vi "Client Data Display.vi"() -> ()   [LabVIEW 2019]
doc: "The Advanced Serial Read and Write example performs a Serial Port Read, a Serial Port Write, or a combination of these actions while setting some advanced serial features like buffer size, termination characters, and XON/XOFF flow control. The user selects the actions (read or write) on the front panel. If both are selected, the VI will write the data first, read the data and then close the VISA session that is opened to the port. \n\nThe parameters set for the serial port must match the parameters of the connected instrument or device. In this example, the bytes to read parameter specifies the number of bytes that the serial port reads. If there were more bytes at the port than the number specified in bytes to read, those bytes would not be read. Also, if you specify to read more bytes than the number of bytes actually read, you might receive a timeout error message.\n\nINSTRUCTIONS:\n1) Select the serial resource and configuration parameters (baud rate, data bits, parity, stop bits, flow control).\n2) Termination character can be enabled and set. Also, set the required input buffer size prior to running the example.\n3) Select the operations to be performed. \n4) Connect the serial port to your device. If no device is available, perform a loopback test by doing one of the following. Short pins 2 and 3 on a RS-232 cable or short pin 4 to pin 8 and pin 5 to pin 9 on a RS-485/422 cable. \n5) Run the VI to see the data read. (The \"read string\" will match the \"string to write\" if a loopback test was performed.)\n\nThis example exposes several advanced features that you may need for your application. Not all applications need all the features shown in this example. The input buffer size is likely an important setting that you want to control in your application. This example expands upon the flow control option for XON and XOFF, allowing the user to choose those control characters. The timeout parameter has been brought to the front panel so a user can specify the time period the VISA Read will wait for the number of bytes to read before timing out. Also, the user has several controls for the termination character, which is discussed later.\n\nNote that you can press the write and read buttons and change the bytes to read parameters on the fly, while the example is running. However, you must stop the example to change the other configuration parameters after the example has started running, and then run again.\n\nSet the I/O buffer size slightly higher the amount of data you expect to receive. This is very important for applications that don't use flow control, as you may lose characters if the receive buffer overflows.\n\nSetting the timeout period ensures that the operation returns with a timeout error if the operation cannot be performed in the specified time period. \n\nSome devices require a termination character in order to identify the end of command strings. Some devices send a termination character to signify the end of data to be read. \n\nThis example shows how you can end the Read operation once a termination character is detected in the buffer and/or append a termination character at the end of the Write data. To enable the Read to end on a termination character, use the VISA Configure Serial Port or use the VISA Properties Serial End Mode for Reads, Termination Character Enable, and Termination Character. To end the Write with a termination character, use the VISA Properties Serial End Mode for Writes, the Send End Enable, and Termination Character. In this example, the same termination character is used for both the Read and the Write. You can specify two different characters for your application, if desired.\n\nYour application may require specific characters for the XON/XOFF Flow Control. You can specify these characters with the VISA Properties Flow Control XOFF Character and Flow Control XON Character. Note that if the standard XON and XOFF characters are used, then decimal 17 and 19 are unavailable for data values. Remember that using flow control and setting an adequate buffer size allow you to prevent buffer overflows."
uses:
  <vilib>/Instr/_visa.llb/VISA Configure Serial Port (Instr).vi
panel:
  out "Output Data":string
  out "Humidity Chart":dbl(graph)
  out "Temperature Chart":dbl(graph)
  out "Humidity":dbl
  out "Temperature":dbl
  out "Actual Bytes Read":u32=47
  in  "Bytes to Read":u32=100
  in  "Stop":bool
  in  "Parity":u16
  in  "Data Bits":u16=8 min=5 max=8 step=1
  in  "Stop Bits":u16=10
  in  "Baud Rate":u32=115200
  in  "VISA Resource Name":refnum<visa-resource-name>="COM10"
  # "Server Serial Port"
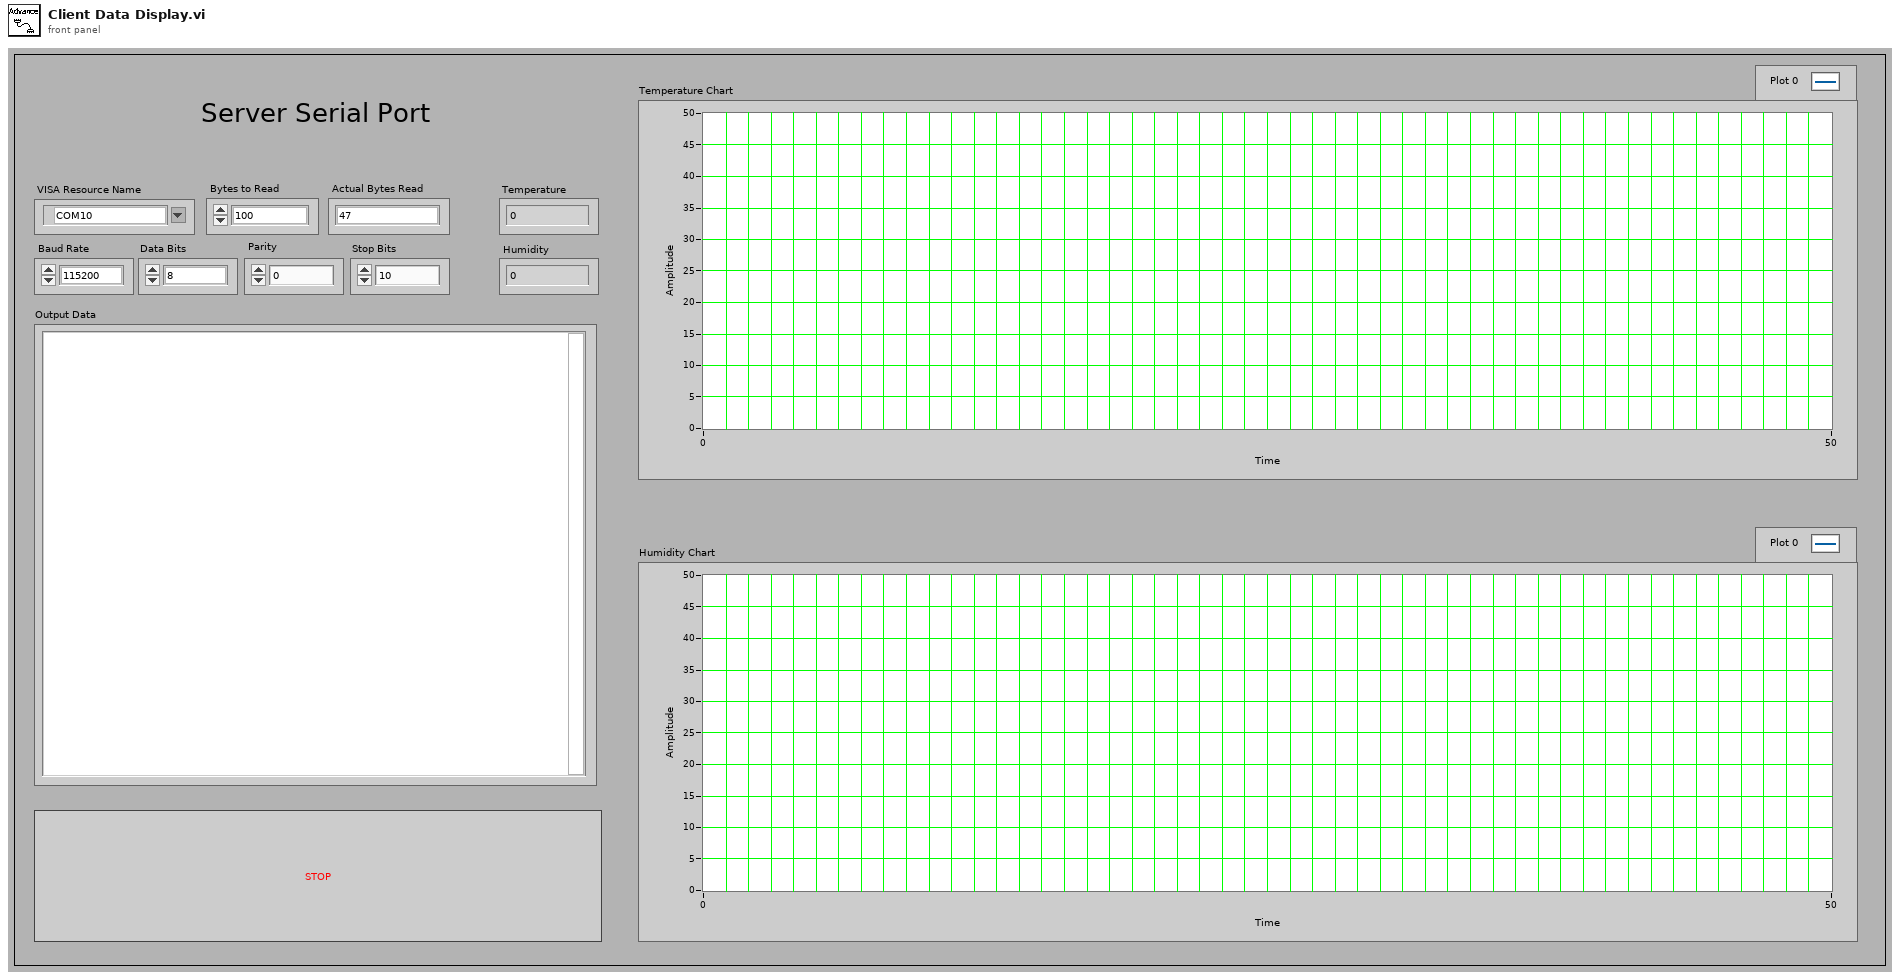
[diagram p1: front panel]
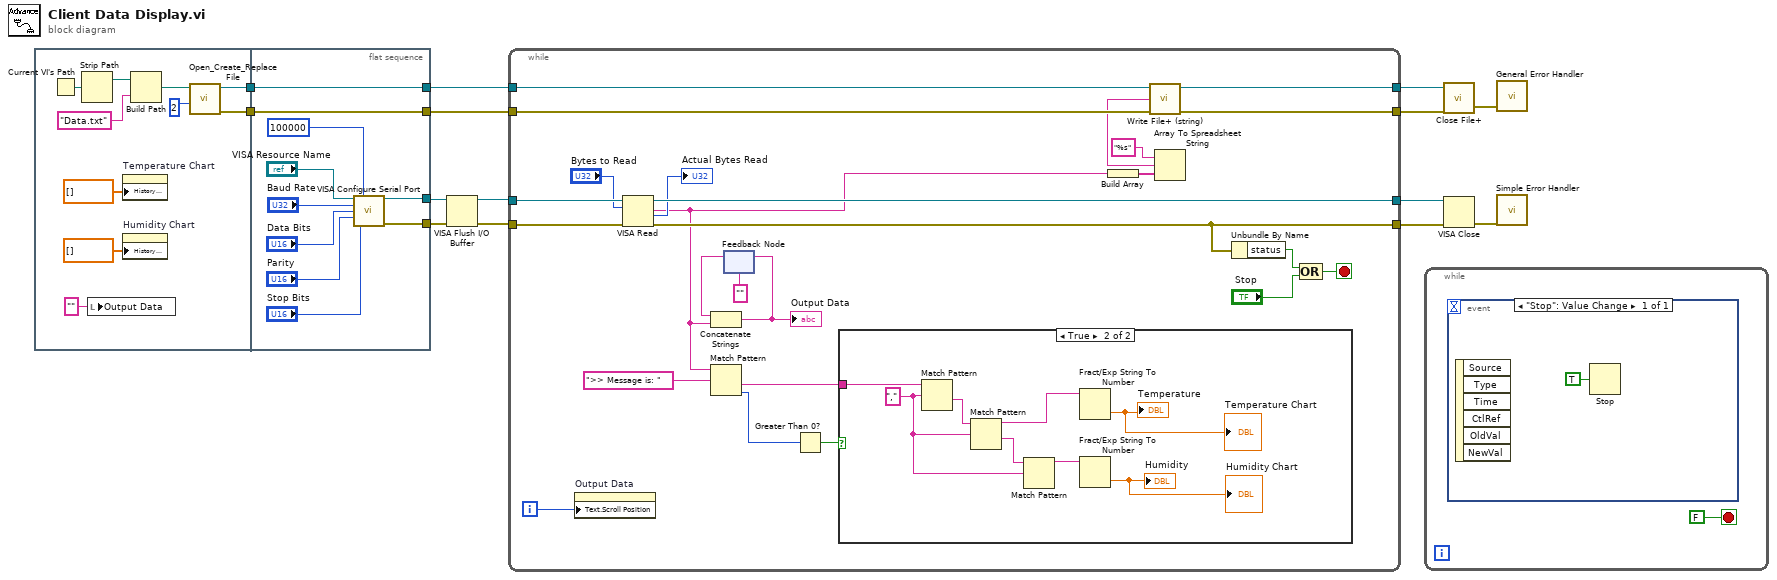
[diagram p0: block diagram]
diagram:
  n1 = flat-sequence {
    tunnel: [w23] -> w6
    tunnel: [w22] -> w5
    tunnel: [w33] -> w9
    tunnel: [w34] -> w10
    tunnel: w6 -> [w34]
    tunnel: w5 -> [w33]
    tunnel: [w27] -> w4
    tunnel: [w26] -> w1
    frame #0 {
      n2 = Current VI's Path() -> (path=w21:path)
      n3 = Strip Path(path=w21) -> (stripped path=w20:path)  [unwired: 1 out]
      n4 = local write "Output Data"("" ("Output Data")) -> ()
      n5 = property on="Temperature Chart" class="WFChart (strict)"("History Data"=dbl[] []) -> ()  [unwired: 2 in, 2 out]
      n6 = property on="Humidity Chart" class="WFChart (strict)"("History Data"=dbl[] []) -> ()  [unwired: 2 in, 2 out]
      n7 = Build Path(base path=w20, name or relative path="Data.txt") -> (appended path=w18:path)
      n8 = call <vilib>:"Open_Create_Replace File.vi"("function (open:0)"=2, "file path"=w18) -> ("error out"=w22:errorcluster, "refnum"=w23:refnum<file>)  [unwired: 4 in, 4 out]
    }
    frame #1 {
      n9 = call-poly "VISA Configure Serial Port"("VISA resource name"="VISA Resource Name", "timeout (10sec)"=u32 100000, "baud rate (9600)"="Baud Rate", "data bits (8)"="Data Bits", "parity (0:none)"="Parity", "stop bits (10: 1 bit)"="Stop Bits") -> ("VISA resource name out"=w27:refnum<visa-resource-name>, "error out"=w26:errorcluster)  [unwired: 4 in, 4 out]
    }
  }
  n10 = VISA Flush I/O Buffer(VISA resource name=w4, error in (no error)=w1) -> (VISA resource name out=w3:refnum<visa-resource-name>, error out=w2:errorcluster)  [unwired: 1 in]
  n11 = while {
    tunnel: w2 -> [w57]
    tunnel: w3 -> [w56]
    tunnel: [w59] -> w13
    tunnel: [w58] -> w12
    tunnel: w10 -> [w50]
    tunnel: w9 -> [w49]
    tunnel: [w51] -> w8
    tunnel: [w52] -> w7
    i -> [w35]
    stop <- w54 stop-if-true
    n12 = property on="Output Data" class="Str"("Text.Scroll Position"=w35) -> ()  [unwired: 2 in, 2 out]
    n13 = VISA Read(VISA resource name=w56, byte count="Bytes to Read", error in (no error)=w57) -> (VISA resource name out=w59:refnum<visa-resource-name>, read buffer=w38:string, return count=→"Actual Bytes Read":u32, error out=w58:errorcluster)
    n14 = Match Pattern(string=w38, regular expression=">> Message is: ") -> (after substring=w39:string, offset past match=w36:i32)  [unwired: 1 in, 2 out]
    n15 = feedback #1("") -> (w46:string)
    n16 = Concatenate Strings(w46, w38) -> (w44:string)
    "Output Data" <- w44
    n17 = feedback-in #1(w44) -> ()
    n18 = Greater Than 0?(x=w36) -> (x > 0?=w37:bool)
    n19 = case shown="True" w37 {
      tunnel: w39 -> [_ w61]
      frame False {
      }
      frame True {
        w60 = "," ("regular expression")
        n20 = Match Pattern(string=w61, regular expression=w60) -> (after substring=w67:string)  [unwired: 1 in, 3 out]
        n21 = Match Pattern(string=w67, regular expression=w60) -> (before substring=w66:string, after substring=w63:string)  [unwired: 1 in, 2 out]
        n22 = Match Pattern(string=w63, regular expression=w60) -> (before substring=w62:string)  [unwired: 1 in, 3 out]
        n23 = Fract/Exp String To Number(string=w66) -> (number=→"Temperature" →"Temperature Chart":dbl)  [unwired: 3 in, 1 out]
        n24 = Fract/Exp String To Number(string=w62) -> (number=→"Humidity" →"Humidity Chart":dbl)  [unwired: 3 in, 1 out]
      }
    }
    n25 = Build Array(w38) -> (w42:string[])
    n26 = Array To Spreadsheet String(array=w42, 3:"%s" ("format string")) -> (spreadsheet string=w40:string)  [unwired: 1 out]
    n27 = call <vilib>:"Write File+ (string).vi"("string"=w40, "error in (no error)"=w49, "refnum"=w50) -> ("error out"=w52:errorcluster, "dup refnum"=w51:refnum<file>)  [unwired: 2 in, 3 out]
    n28 = Unbundle By Name(w58) -> ("status"=w53:bool)
    n29 = Compound Arithmetic op=OR(w53, "Stop") -> (w54:bool)
  }
  n30 = while {
    stop <- FALSE stop-if-true
    n31 = event shown="[0] \"Stop\": Value Change" {
      selector: _ -> [_]
      dyn-events: _ -> [_]
      timeout: _ -> [_]
      event "Stop": Value Change {
        n32 = event-data() -> ()  [unwired: 1 in, 6 out]
        n33 = Stop(stop? (T)=TRUE) -> ()
      }
    }
  }
  n34 = call <vilib>:"Close File+.vi"("error in (no error)"=w7, "refnum"=w8) -> ("error out"=w11:errorcluster)  [unwired: 5 out]
  n35 = VISA Close(VISA resource name=w13, error in (no error)=w12) -> (error out=w14:errorcluster)
  n36 = call <vilib>:"General Error Handler.vi"("error in (no error)"=w11) -> ()  [unwired: 2 in, 13 out]
  n37 = call <vilib>:"Simple Error Handler.vi"("error in (no error)"=w14) -> ()  [unwired: 1 in, 8 out]
